vi "PH_Timing.ProcCases.vi"(0 "i ref in":refnum<vi>, 1 "selector":string, 2 "Data":T1, 3 "call cluster":T2={"Object"="", "Selector"="", "CallType"=enum."synchronous", "Async Object"="", "Async Selector"="", "Data Descriptor"="", "Data"=[], "Error #"=0, "Expire"=0}, 5 "error in (no error)":errorcluster) -> (14 "i ref out":refnum<vi>, 17 "answer cluster":T2={"Object"="", "Selector"="", "CallType"=enum."synchronous", "Async Object"="", "Async Selector"="", "Data Descriptor"="", "Data"=[], "Error #"=0, "Expire"=0}, 19 "error out":errorcluster)   [LabVIEW 2014, in "PH_Timing.lvlib"]
doc: "This method is called by a process from within the default case in the event loop. The methods of a class that are linked to events will be called from THIS method. Add your code here."
uses:
  PH_Timing.lvlib
  CS_Core/CSSystem/CoreDefs/CoreDefs.call_type.ctl
  CS_Core/BaseProcess/BaseProcess.descriptor string definition.ctl
  CS_Core/CSSystem/CoreDefs/CoreDefs.rawDataType.ctl
  PH_Timing.Timing Mode.ctl
  PH_Timing.Slow Trigger Settings.ctl
  PH_Timing.Phase FEs.ctl
  PH_Basics/PH_PowerUnit_BaseClass/PH_PowerUnit_BaseClass.SM States.ctl
  CS_Core/CSSystem/CoreLib/CoreLib.byte array 2 short.vi
  CS_Core/CSSystem/CoreLib/CoreLib.string 2 byte array.vi
  CS_Core/CSSystem/CoreLib/CoreLib.byte array 2 double.vi
  CS_Core/CSSystem/CoreLib/CoreLib.byte array 2 string.vi
  CS_Core/CSSystem/CoreLib/CoreLib.byte array 2 int.vi
  CS_Core/BaseProcess/BaseProcess.lvlib
  CS_Core/CSSystem/CoreLib/CoreLib.lvlib
  CS_Core/CAEObj/CAEObj.lvlib
  PH_Basics/PH_Common/PH_Common.lvlib
  PH_Basics/PH_StatusHandler/PH_StatusHandler.lvlib
  PH_Basics/PH_PowerUnit_BaseClass/PH_PowerUnit_BaseClass.lvlib
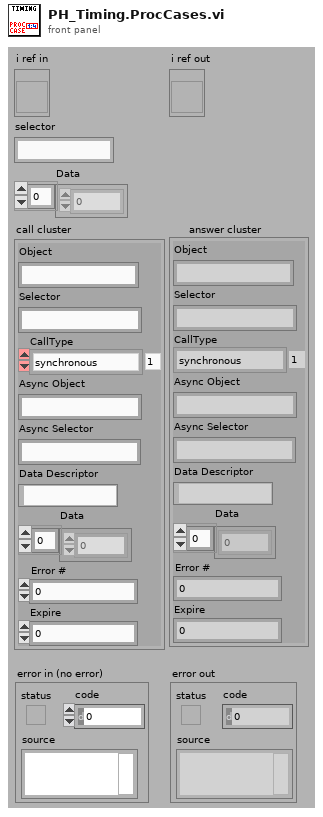
[diagram p1: front panel]
types:
  T1 = typedef "CoreDefs.rawDataType.ctl" = i8[]
  T2 = typedef "CoreDefs.call_type.ctl" = cluster{"Object":string, "Selector":string, "CallType":enum16{"simple", "synchronous", "asynchronous"}, "Async Object":string, "Async Selector":string, "Data Descriptor":T3, "Data":T1, "Error #":i32, "Expire":u32}
  T3 = typedef "BaseProcess.lvlib/BaseProcess.descriptor string definition.ctl" = string
  T4 = typedef "PH_Timing.lvlib/PH_Timing.Timing Mode.ctl" = cluster{"T2":i16, "Modeselector":enum32{"10 Hz", "0.5 Hz", "Shot"}}
  T5 = typedef "PH_Timing.lvlib/PH_Timing.Slow Trigger Settings.ctl" = cluster{"Delay":dbl, "externally triggered?":bool}
  T6 = typedef "PH_Timing.lvlib/PH_Timing.Phase FEs.ctl" = cluster{"Phase":dbl}
  T7 = typedef "PH_PowerUnit_BaseClass.lvlib/PH_PowerUnit_BaseClass.SM States.ctl" = enum16{".", "Stand by", "Switch PU on", "Configure", "Set Default Voltage", "Set STANDBY", "Set READY", "Wait for Shot Cmd", "Open Dump Rods", "Open Ross Relais", "Close Ross Relais", "Switch PSU on", "Switch PSU off", "Charge", "Switch GD Channel on", "Close Dump Rods", "Rods-TO", "RR-TO", "PSU-TO", "Trigger-TO"}
  T8 = typedef "PH_Timing.lvlib/PH_Timing.i attribute.ctl" = cluster{"Sequencer":cluster{"linked?":bool, "Proc State":string, "Ref State":refnum<vi>}, "Gate Generator":cluster{"GD":cluster{"Device Status":T9, "linked?":bool}, "Settings":T10, "GUI Ref":refnum<vi>}, "Interlock Bypass":cluster{"Instancename":string, "Switch linked?":bool, "Device Status":T9, "Ref Status":refnum<vi>}, "Roughtuner":cluster{"Settings":T11, "GUI Ref":refnum<vi>, "GD":cluster{"Device Status":T9, "linked?":bool}}, "0,5Hz Gater":cluster{"Settings":T12, "GUI Ref":refnum<vi>, "GD":cluster{"Device Status":T9, "linked?":bool}}, "Slow Trigger":cluster{"Settings":T5, "GUI Ref":refnum<vi>, "Service ID Delay":i32, "Service ID Ext Trig":i32, "Wanted Settings":T5}, "Timing Mode":cluster{"Mode":T4, "GUI Ref":refnum<vi>, "Service ID T2":i32, "Service ID Mode":i32, "Wanted Mode":T4}, "ns Generator":cluster{"Settings":T13, "ns Generator Settings":refnum<vi>, "GD":cluster{"Device Status":T9, "linked?":bool}}, "Phase FEs":cluster{"Settings":T6, "GUI Ref":refnum<vi>, "Service ID Phase":i32, "Wanted Settings":T6}, "GD GUI Refs":refnum<vi>[], "Heads":T16[], "GUI Ref Delete":refnum<vi>}
  T9 = typedef "PH_StatusHandler.lvlib/PH_StatusHandler.Status.ctl" = i16
  T10 = typedef "PH_Timing.lvlib/PH_Timing.GateGen.ctl" = cluster{"Instance":string, "Channel Gate":i32, "Channel T2":i32, "Width Gate":dbl, "Width T2":dbl, "Delay Gate":dbl, "Delay T2":dbl, "Gate activ":bool, "T2 activ":bool, "System Mode":enum16{"Normal", "Single", "Burst", "Duty Cycle"}}
  T11 = typedef "PH_Timing.lvlib/PH_Timing.Roughtuner.ctl" = cluster{"Instance":string, "Phase PHELIX / UNILAC":cluster{"Channel":u16, "relative to":u16, "Delay [ms]":dbl}, "Pulse Length":cluster{"Channel":u16, "relative to":u16, "Delay [ms]":dbl}, "Trigger":cluster{"externally?":bool, "Rate [Hz]":dbl}}
  T12 = typedef "PH_Timing.lvlib/PH_Timing.0.5HzGater.ctl" = cluster{"Instance":string, "Channel ns FE Delay":i32, "Channel 0.5Hz":i32, "Width ns FE Delay":dbl, "Width 0.5Hz":dbl, "Delay ns FE Delay":dbl, "Delay 0.5Hz":dbl, "ns FE Delay active":bool, "0.5Hz activ":bool, "ns FE Delay inverted":bool, "0.5Hz inverted":bool}
  T13 = typedef "PH_Timing.lvlib/PH_Timing.ns Generator.ctl" = cluster{"Instance":string, "Phase fs / ns FE":cluster{"Channel":T14, "Settings":T15}}
  T14 = typedef "Stanford Research DG645 - Driver.lvlib/Channel.ctl" = i32
  T15 = typedef "PH_SRDG645.lvlib/PH_SRDG645.Channel Settings.ctl" = cluster{"Delay [s]":dbl, "relative to":i32}
  T16 = typedef "PH_Timing.lvlib/PH_Timing.PU Data.ctl" = cluster{"linked?":bool, "Data":T17, "GD":cluster{"Device Status":T9, "linked?":bool}, "GUI Ref":refnum<vi>, "PU":T18}
  T17 = typedef "PH_Timing.lvlib/PH_Timing.PU Info.ctl" = cluster{"Act CH?":bool, "GD":string, "CH":i32, "Delay":dbl, "active":bool, "in Use?":bool}
  T18 = typedef "PH_PP_Common.lvlib/PH_PP_Common.PUs.ctl" = enum16{"no Info", "PA-19mm-1", "PA-19mm-2", "PA-45mm-PILC", "PA-45mm-MAIN", "MA-PU-1", "MA-PU-2", "MA-PU-3", "MA-PU-4", "MA-PU-5", "MA-PU-6", "MA-FR", "MA-PILC", "PA-45mm-DP"}
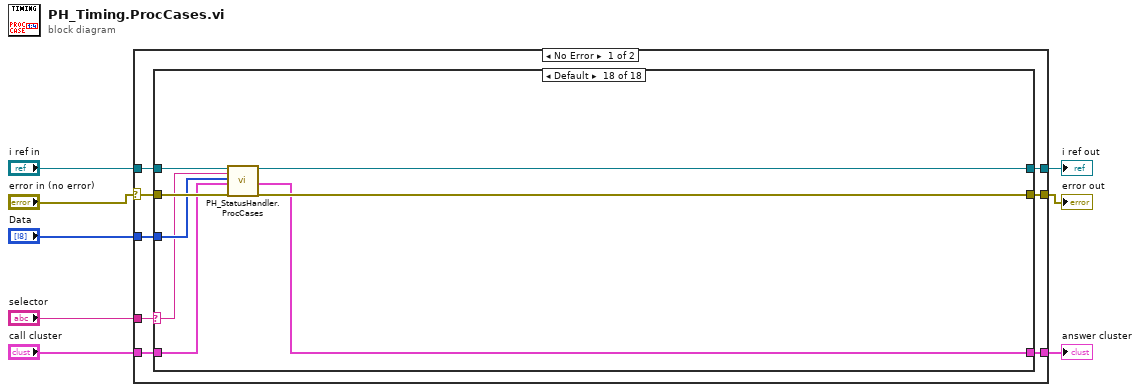
[diagram p0: block diagram]
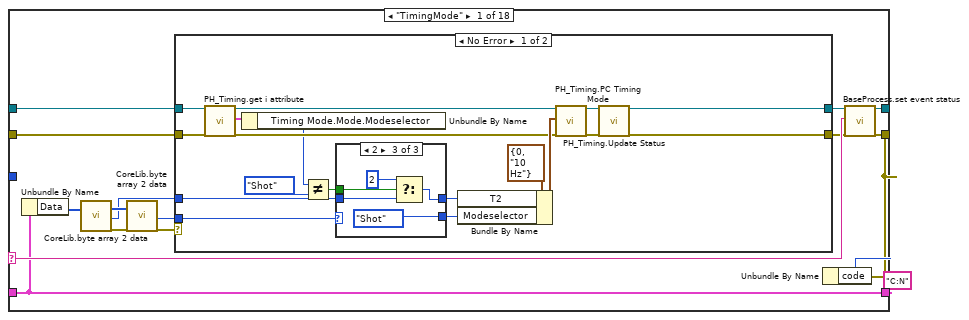
[diagram p2: hidden frame]
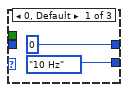
[diagram p3: hidden frame]
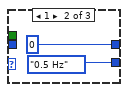
[diagram p4: hidden frame]
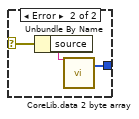
[diagram p6: hidden frame]
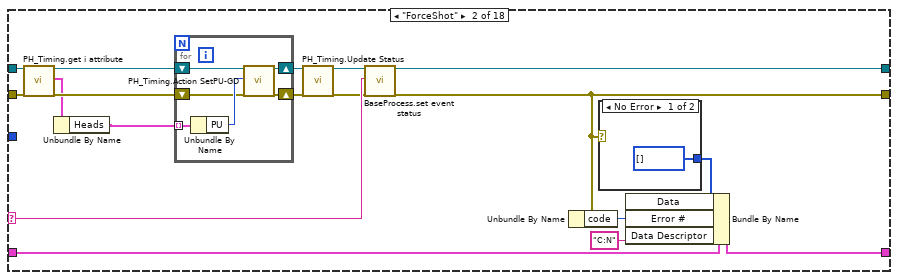
[diagram p7: hidden frame]
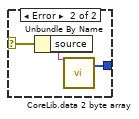
[diagram p8: hidden frame]
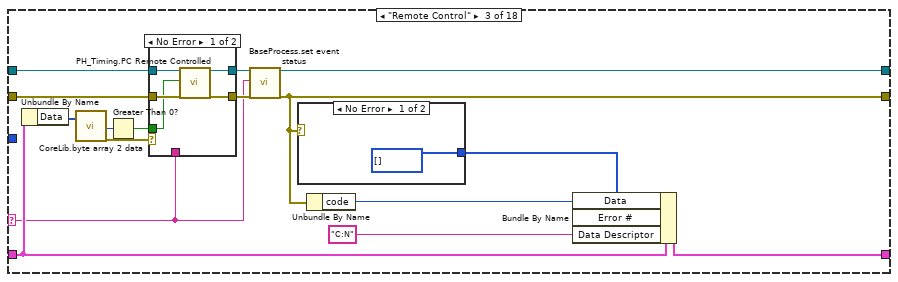
[diagram p9: hidden frame]
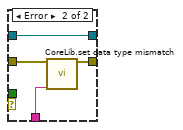
[diagram p10: hidden frame]
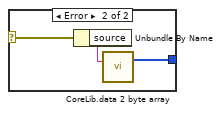
[diagram p11: hidden frame]
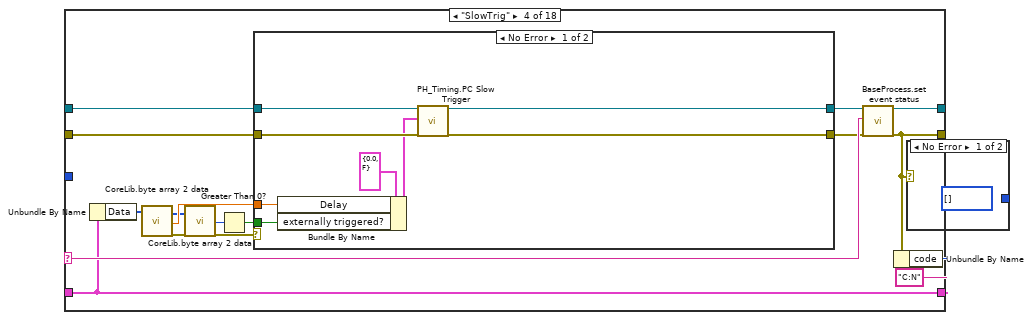
[diagram p12: hidden frame]
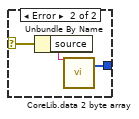
[diagram p14: hidden frame]
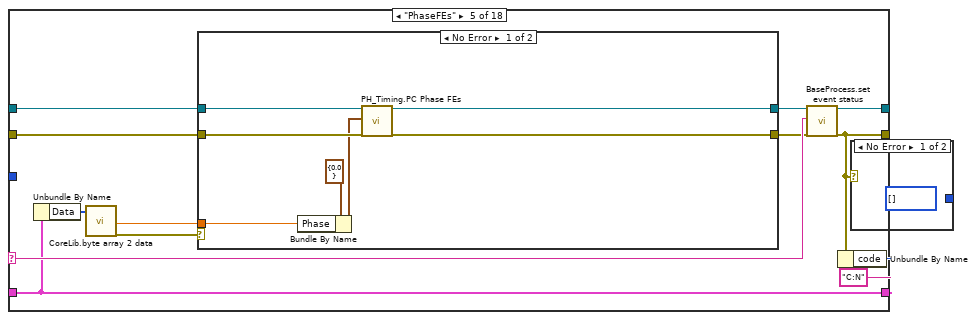
[diagram p15: hidden frame]
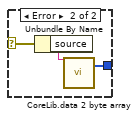
[diagram p17: hidden frame]
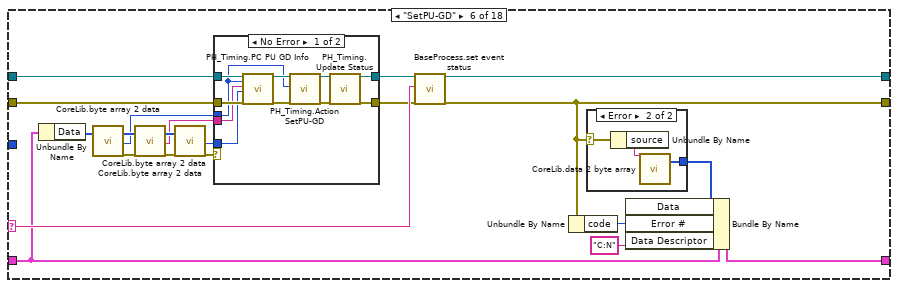
[diagram p18: hidden frame]
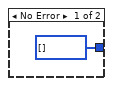
[diagram p20: hidden frame]
diagram:
  n1 = case shown="No Error" "error in (no error)" {
    selector: "error in (no error)" -> [w9 w690]
    tunnel: "selector" -> [w16 _]
    tunnel: [w15 w691] -> w7
    tunnel: "Data" -> [w14 _]
    tunnel: "call cluster" -> [w13 w691]
    tunnel: "i ref in" -> [w12 w692]
    tunnel: [w11 w692] -> w3
    tunnel: [w10 w690] -> w2
    frame No Error {
      n2 = case shown="Default" w16 {
        selector: w16 -> [w28 w79 w96 w137 w166 w200 w235 w267 w317 w351 w386 w444 w500 w534 w568 w602 w641 w683]
        tunnel: w14 -> [_ _ _ _ _ _ _ w259 w311 w345 w378 w436 w494 w528 w562 w594 w633 w684]
        tunnel: w12 -> [w25 w72 w100 w131 w160 w197 w225 w261 w313 w347 w380 w438 w496 w530 w564 w596 w635 w682]
        tunnel: [w30 w81 w107 w139 w168 w202 w237 w270 w320 w354 w389 w447 w503 w537 w571 w605 w630 w689] -> w11
        tunnel: w13 -> [w23 w78 w99 w134 w163 w186 w229 w268 w318 w352 w387 w445 w501 w535 w569 w603 w642 w685]
        tunnel: [w33 w84 w110 w142 w171 w205 w240 w273 w323 w357 w392 w450 w506 w540 w574 w608 w645 w686] -> w15
        tunnel: w9 -> [w24 w71 w101 w132 w161 w196 w226 w260 w312 w346 w379 w437 w495 w529 w563 w595 w634 w688]
        tunnel: [w31 w82 w108 w140 w169 w203 w238 w271 w321 w355 w390 w448 w504 w538 w572 w606 w629 w687] -> w10
        frame "TimingMode" {
          n3 = Unbundle By Name(w23) -> ("Data"=w18:T1)
          n4 = call-poly "CoreLib.byte array 2 data.vi"("byteArray"=w18) -> ("byteArray out"=w20:T1, "i16"=w19:i16, "error out"=w21:errorcluster)  [unwired: 16 in]
          n5 = call-poly "CoreLib.byte array 2 data.vi"("byteArray"=w20, "error in (no error)"=w21) -> ("i16"=w17:i16, "error out"=w22:errorcluster)  [unwired: 15 in, 1 out]
          n6 = case shown="No Error" w22 {
            tunnel: [w37 w63] -> w26
            tunnel: w25 -> [w44 w63]
            tunnel: w24 -> [w52 w62]
            tunnel: [w38 w62] -> w27
            tunnel: w19 -> [w48 _]
            tunnel: w17 -> [w49 _]
            frame No Error {
              n7 = call "PH_Timing.get i attribute.vi"("i ref in"=w44, "error in (no error)"=w52) -> ("i ref out"=w43:refnum<vi>, "i attribute"=w42:T8, "error out"=w45:errorcluster)  [unwired: 15 in]
              n8 = Unbundle By Name(w42) -> ("Timing Mode.Mode.Modeselector"=w41:enum32{"10 Hz", "0.5 Hz", "Shot"})
              n9 = Not Equal?(x=w41, y=enum32{"10 Hz", "0.5 Hz", "Shot"}."Shot") -> (x != y?=w39:bool)
              n10 = case shown="2" w49 {
                tunnel: w48 -> [_ _ w59]
                tunnel: [enum32{"10 Hz", "0.5 Hz", "Shot"}."10 Hz" ("Modeselector") enum32{"10 Hz", "0.5 Hz", "Shot"}."0.5 Hz" ("Modeselector") enum32{"10 Hz", "0.5 Hz", "Shot"}."Shot" ("Modeselector")] -> w47
                tunnel: [i16 0 ("T2 [s]") i16 0 ("T2 [s]") w58] -> w46
                tunnel: w39 -> [_ _ w60]
                frame 0, Default {
                }
                frame 1 {
                }
                frame 2 {
                  n11 = Select(t=i16 2, s=w60, f=w59) -> (s? t:f=w58:i16)
                }
              }
              n12 = Bundle By Name(cluster=T4 {"T2"=0, "Modeselector"=enum."10 Hz"} ("Timing Mode"), "T2"=w46, "Modeselector"=w47) -> (w50:T4)
              n13 = call "PH_Timing.PC Timing Mode.vi"("i ref in"=w43, "Timing Mode"=w50, "error IO"=w45) -> ("i ref out"=w36:refnum<vi>, "error out"=w35:errorcluster)  [unwired: 15 in]
              n14 = call "PH_Timing.Update Status.vi"("i ref in"=w36, "error in (no error)"=w35) -> ("i ref out"=w37:refnum<vi>, "error out"=w38:errorcluster)  [unwired: 16 in]
            }
            frame Error {
            }
          }
          n15 = call "BaseProcess.set event status.vi"("i ref in"=w26, "EventStatus"=w28, "error in (no error)"=w27) -> ("i ref out"=w30:refnum<vi>, "error out"=w31:errorcluster)  [unwired: 14 in, 1 out]
          n16 = Unbundle By Name(w31) -> ("code"=w34:i32)
          n17 = case shown="No Error" w31 {
            selector: w31 -> [_ w67]
            tunnel: [T1 [] ("byteArray out") w66] -> w32
            frame No Error {
            }
            frame Error {
              n18 = Unbundle By Name(w67) -> ("source"=w65:string)
              n19 = call-poly "CoreLib.data 2 byte array.vi"("string"=w65) -> ("byteArray out"=w66:T1)  [unwired: 18 in]
            }
          }
          n20 = Bundle By Name(cluster=w23, "Data"=w32, "Error #"=w34, "Data Descriptor"="C:N") -> (w33:T2)
        }
        frame "ForceShot" {
          n21 = call "PH_Timing.get i attribute.vi"("i ref in"=w72, "error in (no error)"=w71) -> ("i ref out"=w76:refnum<vi>, "i attribute"=w75:T8, "error out"=w77:errorcluster)  [unwired: 15 in]
          n22 = Unbundle By Name(w75) -> ("Heads"=w68:T16[])
          n23 = for {
            shift-right: [w87] -> w73
            shift-left: w76 -> [w89]
            shift-right: [w86] -> w74
            shift-left: w77 -> [w88]
            tunnel: w68 -> [w91] mode=indexing
            n24 = Unbundle By Name(w91) -> ("PU"=w90:T18)
            n25 = call "PH_Timing.Action SetPU-GD.vi"("i ref in"=w89, "PU"=w90, "error in (no error)"=w88) -> ("i ref out"=w87:refnum<vi>, "error out"=w86:errorcluster)  [unwired: 15 in]
          }
          n26 = call "PH_Timing.Update Status.vi"("i ref in"=w73, "error in (no error)"=w74) -> ("i ref out"=w69:refnum<vi>, "error out"=w70:errorcluster)  [unwired: 16 in]
          n27 = call "BaseProcess.set event status.vi"("i ref in"=w69, "EventStatus"=w79, "error in (no error)"=w70) -> ("i ref out"=w81:refnum<vi>, "error out"=w82:errorcluster)  [unwired: 14 in, 1 out]
          n28 = Unbundle By Name(w82) -> ("code"=w85:i32)
          n29 = case shown="No Error" w82 {
            selector: w82 -> [_ w95]
            tunnel: [T1 [] ("byteArray out") w94] -> w83
            frame No Error {
            }
            frame Error {
              n30 = Unbundle By Name(w95) -> ("source"=w93:string)
              n31 = call-poly "CoreLib.data 2 byte array.vi"("string"=w93) -> ("byteArray out"=w94:T1)  [unwired: 18 in]
            }
          }
          n32 = Bundle By Name(cluster=w78, "Data"=w83, "Error #"=w85, "Data Descriptor"="C:N") -> (w84:T2)
        }
        frame "Remote Control" {
          n33 = Unbundle By Name(w99) -> ("Data"=w102:T1)
          n34 = call-poly "CoreLib.byte array 2 data.vi"("byteArray"=w102) -> ("i16"=w103:i16, "error out"=w105:errorcluster)  [unwired: 16 in, 1 out]
          n35 = Greater Than 0?(x=w103) -> (x > 0?=w104:bool)
          n36 = case shown="No Error" w105 {
            tunnel: [w113 w120] -> w98
            tunnel: w100 -> [w115 w120]
            tunnel: w101 -> [w114 w119]
            tunnel: [w116 w118] -> w97
            tunnel: w96 -> [_ w117]
            tunnel: w104 -> [w112 _]
            frame No Error {
              n37 = call "PH_Timing.PC Remote Controlled.vi"("i ref in"=w115, "Remote Controlled?"=w112, "error in (no error)"=w114) -> ("i ref out"=w113:refnum<vi>, "error out"=w116:errorcluster)  [unwired: 15 in]
            }
            frame Error {
              n38 = call "CoreLib.set data type mismatch.vi"("error in (no error)"=w119, "error source"=w117) -> ("error out"=w118:errorcluster)  [unwired: 17 in]
            }
          }
          n39 = call "BaseProcess.set event status.vi"("i ref in"=w98, "EventStatus"=w96, "error in (no error)"=w97) -> ("i ref out"=w107:refnum<vi>, "error out"=w108:errorcluster)  [unwired: 14 in, 1 out]
          n40 = case shown="No Error" w108 {
            selector: w108 -> [_ w124]
            tunnel: [T1 [] ("byteArray out") w123] -> w109
            frame No Error {
            }
            frame Error {
              n41 = Unbundle By Name(w124) -> ("source"=w122:string)
              n42 = call-poly "CoreLib.data 2 byte array.vi"("string"=w122) -> ("byteArray out"=w123:T1)  [unwired: 18 in]
            }
          }
          n43 = Unbundle By Name(w108) -> ("code"=w111:i32)
          n44 = Bundle By Name(cluster=w99, "Data"=w109, "Error #"=w111, "Data Descriptor"="C:N") -> (w110:T2)
        }
        frame "SlowTrig" {
          n45 = Unbundle By Name(w134) -> ("Data"=w130:T1)
          n46 = call-poly "CoreLib.byte array 2 data.vi"("byteArray"=w130) -> ("byteArray out"=w127:T1, "d64"=w133:dbl, "error out"=w129:errorcluster)  [unwired: 16 in]
          n47 = call-poly "CoreLib.byte array 2 data.vi"("byteArray"=w127, "error in (no error)"=w129) -> ("i16"=w126:i16, "error out"=w128:errorcluster)  [unwired: 15 in, 1 out]
          n48 = Greater Than 0?(x=w126) -> (x > 0?=w125:bool)
          n49 = case shown="No Error" w128 {
            tunnel: [w145 w152] -> w135
            tunnel: w132 -> [w150 w153]
            tunnel: [w144 w153] -> w136
            tunnel: w131 -> [w151 w152]
            tunnel: w133 -> [w148 _]
            tunnel: w125 -> [w147 _]
            frame No Error {
              n50 = Bundle By Name(cluster=T5 {"Delay"=0.0, "externally triggered?"=FALSE} ("Slow Trigger Settings"), "Delay"=w148, "externally triggered?"=w147) -> (w146:T5)
              n51 = call "PH_Timing.PC Slow Trigger.vi"("i ref in"=w151, "Slow Trigger Settings"=w146, "error IO"=w150) -> ("i ref out"=w145:refnum<vi>, "error out"=w144:errorcluster)  [unwired: 15 in]
            }
            frame Error {
            }
          }
          n52 = call "BaseProcess.set event status.vi"("i ref in"=w135, "EventStatus"=w137, "error in (no error)"=w136) -> ("i ref out"=w139:refnum<vi>, "error out"=w140:errorcluster)  [unwired: 14 in, 1 out]
          n53 = Unbundle By Name(w140) -> ("code"=w143:i32)
          n54 = case shown="No Error" w140 {
            selector: w140 -> [_ w157]
            tunnel: [T1 [] ("byteArray out") w156] -> w141
            frame No Error {
            }
            frame Error {
              n55 = Unbundle By Name(w157) -> ("source"=w155:string)
              n56 = call-poly "CoreLib.data 2 byte array.vi"("string"=w155) -> ("byteArray out"=w156:T1)  [unwired: 18 in]
            }
          }
          n57 = Bundle By Name(cluster=w134, "Data"=w141, "Error #"=w143, "Data Descriptor"="C:N") -> (w142:T2)
        }
        frame "PhaseFEs" {
          n58 = Unbundle By Name(w163) -> ("Data"=w159:T1)
          n59 = call-poly "CoreLib.byte array 2 data.vi"("byteArray"=w159) -> ("d64"=w162:dbl, "error out"=w158:errorcluster)  [unwired: 16 in, 1 out]
          n60 = case shown="No Error" w158 {
            tunnel: [w175 w180] -> w164
            tunnel: w161 -> [w178 w181]
            tunnel: [w174 w181] -> w165
            tunnel: w160 -> [w179 w180]
            tunnel: w162 -> [w176 _]
            frame No Error {
              n61 = Bundle By Name(cluster=T6 {"Phase"=0.0} ("FE Phase"), "Phase"=w176) -> (w173:T6)
              n62 = call "PH_Timing.PC Phase FEs.vi"("i ref in"=w179, "FE Phase"=w173, "error IO"=w178) -> ("i ref out"=w175:refnum<vi>, "error out"=w174:errorcluster)  [unwired: 15 in]
            }
            frame Error {
            }
          }
          n63 = call "BaseProcess.set event status.vi"("i ref in"=w164, "EventStatus"=w166, "error in (no error)"=w165) -> ("i ref out"=w168:refnum<vi>, "error out"=w169:errorcluster)  [unwired: 14 in, 1 out]
          n64 = Unbundle By Name(w169) -> ("code"=w172:i32)
          n65 = case shown="No Error" w169 {
            selector: w169 -> [_ w185]
            tunnel: [T1 [] ("byteArray out") w184] -> w170
            frame No Error {
            }
            frame Error {
              n66 = Unbundle By Name(w185) -> ("source"=w183:string)
              n67 = call-poly "CoreLib.data 2 byte array.vi"("string"=w183) -> ("byteArray out"=w184:T1)  [unwired: 18 in]
            }
          }
          n68 = Bundle By Name(cluster=w163, "Data"=w170, "Error #"=w172, "Data Descriptor"="C:N") -> (w171:T2)
        }
        frame "SetPU-GD" {
          n69 = Unbundle By Name(w186) -> ("Data"=w195:T1)
          n70 = call-poly "CoreLib.byte array 2 data.vi"("byteArray"=w195) -> ("byteArray out"=w193:T1, "i16"=w189:i16, "error out"=w194:errorcluster)  [unwired: 16 in]
          n71 = call-poly "CoreLib.byte array 2 data.vi"("byteArray"=w193, "error in (no error)"=w194) -> ("byteArray out"=w190:T1, "string"=w188:string, "error out"=w192:errorcluster)  [unwired: 15 in]
          n72 = call-poly "CoreLib.byte array 2 data.vi"("byteArray"=w190, "error in (no error)"=w192) -> ("i32"=w187:i32, "error out"=w191:errorcluster)  [unwired: 15 in, 1 out]
          n73 = case shown="No Error" w191 {
            tunnel: [w208 w219] -> w198
            tunnel: w197 -> [w217 w219]
            tunnel: w196 -> [w216 w218]
            tunnel: [w209 w218] -> w199
            tunnel: w189 -> [w207 _]
            tunnel: w188 -> [w215 _]
            tunnel: w187 -> [w212 _]
            frame No Error {
              n74 = call "PH_Timing.PC PU GD Info.vi"("i ref in"=w217, "PU"=w207, "GD Instance Name"=w215, "PU Channel"=w212, "error in"=w216) -> ("i ref out"=w211:refnum<vi>, "error out"=w210:errorcluster)  [unwired: 13 in]
              n75 = call "PH_Timing.Action SetPU-GD.vi"("i ref in"=w211, "PU"=w207, "error in (no error)"=w210) -> ("i ref out"=w214:refnum<vi>, "error out"=w213:errorcluster)  [unwired: 15 in]
              n76 = call "PH_Timing.Update Status.vi"("i ref in"=w214, "error in (no error)"=w213) -> ("i ref out"=w208:refnum<vi>, "error out"=w209:errorcluster)  [unwired: 16 in]
            }
            frame Error {
            }
          }
          n77 = call "BaseProcess.set event status.vi"("i ref in"=w198, "EventStatus"=w200, "error in (no error)"=w199) -> ("i ref out"=w202:refnum<vi>, "error out"=w203:errorcluster)  [unwired: 14 in, 1 out]
          n78 = Unbundle By Name(w203) -> ("code"=w206:i32)
          n79 = case shown="Error" w203 {
            selector: w203 -> [_ w223]
            tunnel: [T1 [] ("byteArray out") w222] -> w204
            frame No Error {
            }
            frame Error {
              n80 = Unbundle By Name(w223) -> ("source"=w221:string)
              n81 = call-poly "CoreLib.data 2 byte array.vi"("string"=w221) -> ("byteArray out"=w222:T1)  [unwired: 18 in]
            }
          }
          n82 = Bundle By Name(cluster=w186, "Data"=w204, "Error #"=w206, "Data Descriptor"="C:N") -> (w205:T2)
        }
        frame "SetPUDelay" {
          n83 = Unbundle By Name(w229) -> ("Data"=w232:T1)
          n84 = call-poly "CoreLib.byte array 2 data.vi"("byteArray"=w232) -> ("byteArray out"=w228:T1, "i16"=w224:i16, "error out"=w231:errorcluster)  [unwired: 16 in]
          n85 = call-poly "CoreLib.byte array 2 data.vi"("byteArray"=w228, "error in (no error)"=w231) -> ("d64"=w227:dbl, "error out"=w230:errorcluster)  [unwired: 15 in, 1 out]
          n86 = case shown="No Error" w230 {
            tunnel: [w243 w252] -> w233
            tunnel: w226 -> [w251 w253]
            tunnel: [w246 w253] -> w234
            tunnel: w225 -> [w249 w252]
            tunnel: w227 -> [w250 _]
            tunnel: w224 -> [w242 _]
            frame No Error {
              n87 = call "PH_Timing.PC PU Delay.vi"("i ref in"=w249, "PU"=w242, "PU Delay"=w250, "error in"=w251) -> ("i ref out"=w244:refnum<vi>, "error out"=w247:errorcluster)  [unwired: 14 in]
              n88 = call "PH_Timing.Action SetPU-GD.vi"("i ref in"=w244, "PU"=w242, "error in (no error)"=w247) -> ("i ref out"=w245:refnum<vi>, "error out"=w248:errorcluster)  [unwired: 15 in]
              n89 = call "PH_Timing.Update Status.vi"("i ref in"=w245, "error in (no error)"=w248) -> ("i ref out"=w243:refnum<vi>, "error out"=w246:errorcluster)  [unwired: 16 in]
            }
            frame Error {
            }
          }
          n90 = call "BaseProcess.set event status.vi"("i ref in"=w233, "EventStatus"=w235, "error in (no error)"=w234) -> ("i ref out"=w237:refnum<vi>, "error out"=w238:errorcluster)  [unwired: 14 in, 1 out]
          n91 = Unbundle By Name(w238) -> ("code"=w241:i32)
          n92 = case shown="No Error" w238 {
            selector: w238 -> [_ w257]
            tunnel: [T1 [] ("byteArray out") w256] -> w239
            frame No Error {
            }
            frame Error {
              n93 = Unbundle By Name(w257) -> ("source"=w255:string)
              n94 = call-poly "CoreLib.data 2 byte array.vi"("string"=w255) -> ("byteArray out"=w256:T1)  [unwired: 18 in]
            }
          }
          n95 = Bundle By Name(cluster=w229, "Data"=w239, "Error #"=w241, "Data Descriptor"="C:N") -> (w240:T2)
        }
        frame "_StatusInterlockSwitch" {
          n96 = call "CAEObj.unfold trend data.vi"("i ref in"=w261, "raw trend data"=w259) -> ("no link"=w265:bool, "data"=w264:i8[], "typeDescriptor"=w258:string, "error out"=w266:errorcluster)  [unwired: 9 in, 5 out]
          n97 = case shown="No Error" w266 {
            tunnel: [w293 w302] -> w262
            tunnel: w261 -> [w287 w302]
            tunnel: w260 -> [w289 w301]
            tunnel: [w294 w301] -> w263
            tunnel: w265 -> [w276 _]
            tunnel: w264 -> [w292 _]
            tunnel: w258 -> [w290 _]
            frame No Error {
              n98 = call "PH_Timing.get i attribute.vi"("i ref in"=w287, "error in (no error)"=w289) -> ("i ref out"=w286:refnum<vi>, "i attribute"=w281:T8, "error out"=w288:errorcluster)  [unwired: 15 in]
              n99 = call "PH_StatusHandler.get Status DIM Service.vi"("no link"=w276, "typeDescriptor"=w290, "data"=w292) -> ("Status"=w291:T9)  [unwired: 1 in]
              n100 = Unbundle By Name(w281) -> ("Interlock Bypass.Switch linked?"=w280:bool)
              n101 = Not(x=w276) -> (.not. x?=w275:bool)
              n102 = call "PH_Timing.PC Status Interlockswitch.vi"("i ref in"=w286, "IL Switch Status"=w291, "no link"=w276, "error in"=w288) -> ("i ref out"=w285:refnum<vi>, "error out"=w283:errorcluster)  [unwired: 14 in]
              n103 = Bundle("Switch linked?"=w280, w275) -> (w279:cluster{"Switch linked?":bool, bool})  [unwired: 1 in]
              n104 = Equal?(x=w279, y=cluster{"linked?":bool, "no link":bool} {"linked?"=FALSE, "no link"=TRUE}) -> (x = y?=w277:bool)
              n105 = case shown="True" w277 {
                tunnel: w285 -> [w296 w300]
                tunnel: [w296 w299] -> w284
                tunnel: w283 -> [w295 w298]
                tunnel: [w295 w297] -> w282
                frame False {
                }
                frame True {
                  n106 = call "PH_Timing.Action Switch Interlock Bypass.vi"("i ref in"=w300, "error in (no error)"=w298) -> ("i ref out"=w299:refnum<vi>, "error out"=w297:errorcluster)  [unwired: 16 in]
                }
              }
              n107 = call "PH_Timing.Update Status.vi"("i ref in"=w284, "error in (no error)"=w282) -> ("i ref out"=w293:refnum<vi>, "error out"=w294:errorcluster)  [unwired: 16 in]
            }
            frame Error {
            }
          }
          n108 = call "BaseProcess.set event status.vi"("i ref in"=w262, "EventStatus"=w267, "error in (no error)"=w263) -> ("i ref out"=w270:refnum<vi>, "error out"=w271:errorcluster)  [unwired: 14 in, 1 out]
          n109 = Unbundle By Name(w271) -> ("code"=w274:i32)
          n110 = case shown="No Error" w271 {
            selector: w271 -> [_ w306]
            tunnel: [T1 [] ("byteArray out") w305] -> w272
            frame No Error {
            }
            frame Error {
              n111 = Unbundle By Name(w306) -> ("source"=w304:string)
              n112 = call-poly "CoreLib.data 2 byte array.vi"("string"=w304) -> ("byteArray out"=w305:T1)  [unwired: 18 in]
            }
          }
          n113 = Bundle By Name(cluster=w268, "Data"=w272, "Error #"=w274, "Data Descriptor"="C:N") -> (w273:T2)
        }
        frame "_linkBNCChannelInfo" {
          n114 = call "CAEObj.unfold trend data.vi"("i ref in"=w313, "raw trend data"=w311) -> ("no link"=w315:bool, "data"=w314:i8[], "serviceName"=w310:string, "typeDescriptor"=w309:string, "error out"=w316:errorcluster)  [unwired: 9 in, 4 out]
          n115 = case shown="No Error" w316 {
            tunnel: [w327 w336] -> w308
            tunnel: w313 -> [w333 w336]
            tunnel: w312 -> [w334 w335]
            tunnel: [w325 w335] -> w307
            tunnel: w315 -> [w332 _]
            tunnel: w314 -> [w331 _]
            tunnel: w310 -> [w330 _]
            tunnel: w309 -> [w329 _]
            frame No Error {
              n116 = call "PH_Timing.PC link BNC Channel Infos.vi"("i ref in"=w333, "data"=w331, "Service Name"=w330, "typeDescriptor"=w329, "no link"=w332, "error in"=w334) -> ("i ref out"=w328:refnum<vi>, "error out"=w326:errorcluster)  [unwired: 12 in]
              n117 = call "PH_Timing.Update Status.vi"("i ref in"=w328, "error in (no error)"=w326) -> ("i ref out"=w327:refnum<vi>, "error out"=w325:errorcluster)  [unwired: 16 in]
            }
            frame Error {
            }
          }
          n118 = call "BaseProcess.set event status.vi"("i ref in"=w308, "EventStatus"=w317, "error in (no error)"=w307) -> ("i ref out"=w320:refnum<vi>, "error out"=w321:errorcluster)  [unwired: 14 in, 1 out]
          n119 = Unbundle By Name(w321) -> ("code"=w324:i32)
          n120 = case shown="No Error" w321 {
            selector: w321 -> [_ w340]
            tunnel: [T1 [] ("byteArray out") w339] -> w322
            frame No Error {
            }
            frame Error {
              n121 = Unbundle By Name(w340) -> ("source"=w338:string)
              n122 = call-poly "CoreLib.data 2 byte array.vi"("string"=w338) -> ("byteArray out"=w339:T1)  [unwired: 18 in]
            }
          }
          n123 = Bundle By Name(cluster=w318, "Data"=w322, "Error #"=w324, "Data Descriptor"="C:N") -> (w323:T2)
        }
        frame "_linkBNCSysModeInfo" {
          n124 = call "CAEObj.unfold trend data.vi"("i ref in"=w347, "raw trend data"=w345) -> ("no link"=w349:bool, "data"=w348:i8[], "serviceName"=w344:string, "typeDescriptor"=w343:string, "error out"=w350:errorcluster)  [unwired: 9 in, 4 out]
          n125 = case shown="No Error" w350 {
            tunnel: [w361 w370] -> w342
            tunnel: w347 -> [w367 w370]
            tunnel: w346 -> [w368 w369]
            tunnel: [w359 w369] -> w341
            tunnel: w349 -> [w366 _]
            tunnel: w348 -> [w365 _]
            tunnel: w344 -> [w364 _]
            tunnel: w343 -> [w363 _]
            frame No Error {
              n126 = call "PH_Timing.PC link BNC System Mode Infos.vi"("i ref in"=w367, "data"=w365, "Service Name"=w364, "typeDescriptor"=w363, "no link"=w366, "error in"=w368) -> ("i ref out"=w362:refnum<vi>, "error out"=w360:errorcluster)  [unwired: 12 in]
              n127 = call "PH_Timing.Update Status.vi"("i ref in"=w362, "error in (no error)"=w360) -> ("i ref out"=w361:refnum<vi>, "error out"=w359:errorcluster)  [unwired: 16 in]
            }
            frame Error {
            }
          }
          n128 = call "BaseProcess.set event status.vi"("i ref in"=w342, "EventStatus"=w351, "error in (no error)"=w341) -> ("i ref out"=w354:refnum<vi>, "error out"=w355:errorcluster)  [unwired: 14 in, 1 out]
          n129 = Unbundle By Name(w355) -> ("code"=w358:i32)
          n130 = case shown="No Error" w355 {
            selector: w355 -> [_ w374]
            tunnel: [T1 [] ("byteArray out") w373] -> w356
            frame No Error {
            }
            frame Error {
              n131 = Unbundle By Name(w374) -> ("source"=w372:string)
              n132 = call-poly "CoreLib.data 2 byte array.vi"("string"=w372) -> ("byteArray out"=w373:T1)  [unwired: 18 in]
            }
          }
          n133 = Bundle By Name(cluster=w352, "Data"=w356, "Error #"=w358, "Data Descriptor"="C:N") -> (w357:T2)
        }
        frame "_activateCHs" {
          n134 = call "CAEObj.unfold trend data.vi"("i ref in"=w380, "raw trend data"=w378) -> ("quality"=w375:i32, "no link"=w384:bool, "data"=w383:i8[], "serviceName"=w377:string, "typeDescriptor"=w376:string, "error out"=w385:errorcluster)  [unwired: 9 in, 3 out]
          n135 = case shown="No Error" w385 {
            tunnel: [w403 w428] -> w381
            tunnel: w380 -> [w406 w428]
            tunnel: w379 -> [w405 w427]
            tunnel: [w404 w427] -> w382
            tunnel: w384 -> [w402 _]
            tunnel: w383 -> [w411 _]
            tunnel: w377 -> [w409 _]
            tunnel: w376 -> [w412 _]
            tunnel: w375 -> [w410 _]
            frame No Error {
              n136 = call "PH_DIM.get String.vi"("no link"=w402, "typeDescriptor"=w412, "data"=w411, "quality"=w410) -> ("Output String"=w397:string)
              n137 = call "PH_Strings.Remove trailing Zeros.vi"("Input String"=w397) -> ("Output String"=w396:string)
              n138 = call "PH_PowerUnit_BaseClass.String to SM State.vi"("SM State String"=w396) -> ("SM State"=w395:T7)
              n139 = Equal?(x=w395, y=PH_PowerUnit_BaseClass.SM_States."Switch GD Channel on" ("SM State")) -> (x = y?=w398:bool)
              n140 = call "PH_Timing.PC activate CHs.vi"("i ref in"=w406, "Service Name"=w409, "Activate CH?"=w398, "no link"=w402, "error in"=w405) -> ("i ref out"=w408:refnum<vi>, "PU"=w401:T18, "error out"=w407:errorcluster)  [unwired: 12 in]
              n141 = case shown="False" w402 {
                tunnel: w408 -> [w417 w426]
                tunnel: [w414 w426] -> w400
                tunnel: w407 -> [w416 w425]
                tunnel: [w415 w425] -> w399
                tunnel: w401 -> [w413 _]
                frame False {
                  n142 = case shown="Default" w413 {
                    selector: w413 -> [_ w420]
                    tunnel: w417 -> [w419 w424]
                    tunnel: w416 -> [w418 w423]
                    tunnel: [w418 w422] -> w415
                    tunnel: [w419 w421] -> w414
                    frame "no Info" {
                    }
                    frame Default {
                      n143 = call "PH_Timing.Action link PUs.vi"("i ref in"=w424, "PU index"=w420, "error in (no error)"=w423) -> ("i ref out"=w421:refnum<vi>, "error out"=w422:errorcluster)  [unwired: 15 in]
                    }
                  }
                }
                frame True {
                }
              }
              n144 = call "PH_Timing.Update Status.vi"("i ref in"=w400, "error in (no error)"=w399) -> ("i ref out"=w403:refnum<vi>, "error out"=w404:errorcluster)  [unwired: 16 in]
            }
            frame Error {
            }
          }
          n145 = call "BaseProcess.set event status.vi"("i ref in"=w381, "EventStatus"=w386, "error in (no error)"=w382) -> ("i ref out"=w389:refnum<vi>, "error out"=w390:errorcluster)  [unwired: 14 in, 1 out]
          n146 = Unbundle By Name(w390) -> ("code"=w393:i32)
          n147 = case shown="No Error" w390 {
            selector: w390 -> [_ w432]
            tunnel: [T1 [] ("byteArray out") w431] -> w391
            frame No Error {
            }
            frame Error {
              n148 = Unbundle By Name(w432) -> ("source"=w430:string)
              n149 = call-poly "CoreLib.data 2 byte array.vi"("string"=w430) -> ("byteArray out"=w431:T1)  [unwired: 18 in]
            }
          }
          n150 = Bundle By Name(cluster=w387, "Data"=w391, "Error #"=w393, "Data Descriptor"="C:N") -> (w392:T2)
        }
        frame "_PUsinUse" {
          n151 = call "CAEObj.unfold trend data.vi"("i ref in"=w438, "raw trend data"=w436) -> ("quality"=w434:i32, "no link"=w442:bool, "data"=w441:i8[], "serviceName"=w433:string, "typeDescriptor"=w435:string, "error out"=w443:errorcluster)  [unwired: 9 in, 3 out]
          n152 = case shown="No Error" w443 {
            tunnel: [w464 w485] -> w439
            tunnel: w438 -> [w461 w485]
            tunnel: w437 -> [w460 w484]
            tunnel: [w465 w484] -> w440
            tunnel: w442 -> [w452 _]
            tunnel: w441 -> [w467 _]
            tunnel: w435 -> [w468 _]
            tunnel: w434 -> [w466 _]
            tunnel: w433 -> [w459 _]
            frame No Error {
              n153 = call "PH_DIM.get Boolean.vi"("no link"=w452, "typeDescriptor"=w468, "data"=w467, "quality"=w466) -> ("Value"=w463:i32)
              n154 = Equal?(x=2, y=w463) -> (x = y?=w458:bool)
              n155 = call "PH_Timing.PC PU in Use.vi"("i ref in"=w461, "Service Name"=w459, "PU in Use?"=w458, "no link?"=w452, "error in"=w460) -> ("i ref out"=w456:refnum<vi>, "PU"=w453:T18, "error out"=w457:errorcluster)  [unwired: 12 in]
              n156 = case shown="Default" w453 {
                selector: w453 -> [_ w471]
                tunnel: w456 -> [w470 w475]
                tunnel: w457 -> [w469 w474]
                tunnel: [w470 w473] -> w455
                tunnel: [w469 w472] -> w454
                frame "no Info" {
                }
                frame Default {
                  n157 = call "PH_Timing.Action SetPU-GD.vi"("i ref in"=w475, "PU"=w471, "error in (no error)"=w474) -> ("i ref out"=w473:refnum<vi>, "error out"=w472:errorcluster)  [unwired: 15 in]
                }
              }
              n158 = case shown="\"MA-FR\"" w453 {
                tunnel: [w476 w483] -> w465
                tunnel: [w477 w482] -> w464
                tunnel: w455 -> [w477 w479]
                tunnel: w454 -> [w476 w478]
                frame Default {
                }
                frame "MA-FR" {
                  n159 = call "PH_Timing.Action Switch Interlock Bypass.vi"("i ref in"=w479, "error in (no error)"=w478) -> ("i ref out"=w481:refnum<vi>, "error out"=w480:errorcluster)  [unwired: 16 in]
                  n160 = call "PH_Timing.Update Status.vi"("i ref in"=w481, "error in (no error)"=w480) -> ("i ref out"=w482:refnum<vi>, "error out"=w483:errorcluster)  [unwired: 16 in]
                }
              }
            }
            frame Error {
            }
          }
          n161 = call "BaseProcess.set event status.vi"("i ref in"=w439, "EventStatus"=w444, "error in (no error)"=w440) -> ("i ref out"=w447:refnum<vi>, "error out"=w448:errorcluster)  [unwired: 14 in, 1 out]
          n162 = Unbundle By Name(w448) -> ("code"=w451:i32)
          n163 = case shown="No Error" w448 {
            selector: w448 -> [_ w489]
            tunnel: [T1 [] ("byteArray out") w488] -> w449
            frame No Error {
            }
            frame Error {
              n164 = Unbundle By Name(w489) -> ("source"=w487:string)
              n165 = call-poly "CoreLib.data 2 byte array.vi"("string"=w487) -> ("byteArray out"=w488:T1)  [unwired: 18 in]
            }
          }
          n166 = Bundle By Name(cluster=w445, "Data"=w449, "Error #"=w451, "Data Descriptor"="C:N") -> (w450:T2)
        }
        frame "_linkSRDGChannelInfo" {
          n167 = call "CAEObj.unfold trend data.vi"("i ref in"=w496, "raw trend data"=w494) -> ("no link"=w498:bool, "data"=w497:i8[], "serviceName"=w493:string, "typeDescriptor"=w492:string, "error out"=w499:errorcluster)  [unwired: 9 in, 4 out]
          n168 = case shown="No Error" w499 {
            tunnel: [w510 w519] -> w491
            tunnel: w496 -> [w516 w519]
            tunnel: w495 -> [w517 w518]
            tunnel: [w508 w518] -> w490
            tunnel: w498 -> [w515 _]
            tunnel: w497 -> [w514 _]
            tunnel: w493 -> [w513 _]
            tunnel: w492 -> [w512 _]
            frame No Error {
              n169 = call "PH_Timing.PC link SRDG Channel Infos.vi"("i ref in"=w516, "data"=w514, "Service Name"=w513, "typeDescriptor"=w512, "no link"=w515, "error in"=w517) -> ("i ref out"=w511:refnum<vi>, "error out"=w509:errorcluster)  [unwired: 12 in]
              n170 = call "PH_Timing.Update Status.vi"("i ref in"=w511, "error in (no error)"=w509) -> ("i ref out"=w510:refnum<vi>, "error out"=w508:errorcluster)  [unwired: 16 in]
            }
            frame Error {
            }
          }
          n171 = call "BaseProcess.set event status.vi"("i ref in"=w491, "EventStatus"=w500, "error in (no error)"=w490) -> ("i ref out"=w503:refnum<vi>, "error out"=w504:errorcluster)  [unwired: 14 in, 1 out]
          n172 = Unbundle By Name(w504) -> ("code"=w507:i32)
          n173 = case shown="No Error" w504 {
            selector: w504 -> [_ w523]
            tunnel: [T1 [] ("byteArray out") w522] -> w505
            frame No Error {
            }
            frame Error {
              n174 = Unbundle By Name(w523) -> ("source"=w521:string)
              n175 = call-poly "CoreLib.data 2 byte array.vi"("string"=w521) -> ("byteArray out"=w522:T1)  [unwired: 18 in]
            }
          }
          n176 = Bundle By Name(cluster=w501, "Data"=w505, "Error #"=w507, "Data Descriptor"="C:N") -> (w506:T2)
        }
        frame "_linkSRDGRatelInfo" {
          n177 = call "CAEObj.unfold trend data.vi"("i ref in"=w530, "raw trend data"=w528) -> ("no link"=w532:bool, "data"=w531:i8[], "serviceName"=w527:string, "typeDescriptor"=w526:string, "error out"=w533:errorcluster)  [unwired: 9 in, 4 out]
          n178 = case shown="No Error" w533 {
            tunnel: [w544 w553] -> w525
            tunnel: w530 -> [w550 w553]
            tunnel: w529 -> [w551 w552]
            tunnel: [w542 w552] -> w524
            tunnel: w532 -> [w549 _]
            tunnel: w531 -> [w548 _]
            tunnel: w527 -> [w547 _]
            tunnel: w526 -> [w546 _]
            frame No Error {
              n179 = call "PH_Timing.PC link SRDG Rate Info.vi"("i ref in"=w550, "data"=w548, "Service Name"=w547, "typeDescriptor"=w546, "no link"=w549, "error in"=w551) -> ("i ref out"=w545:refnum<vi>, "error out"=w543:errorcluster)  [unwired: 12 in]
              n180 = call "PH_Timing.Update Status.vi"("i ref in"=w545, "error in (no error)"=w543) -> ("i ref out"=w544:refnum<vi>, "error out"=w542:errorcluster)  [unwired: 16 in]
            }
            frame Error {
            }
          }
          n181 = call "BaseProcess.set event status.vi"("i ref in"=w525, "EventStatus"=w534, "error in (no error)"=w524) -> ("i ref out"=w537:refnum<vi>, "error out"=w538:errorcluster)  [unwired: 14 in, 1 out]
          n182 = Unbundle By Name(w538) -> ("code"=w541:i32)
          n183 = case shown="No Error" w538 {
            selector: w538 -> [_ w557]
            tunnel: [T1 [] ("byteArray out") w556] -> w539
            frame No Error {
            }
            frame Error {
              n184 = Unbundle By Name(w557) -> ("source"=w555:string)
              n185 = call-poly "CoreLib.data 2 byte array.vi"("string"=w555) -> ("byteArray out"=w556:T1)  [unwired: 18 in]
            }
          }
          n186 = Bundle By Name(cluster=w535, "Data"=w539, "Error #"=w541, "Data Descriptor"="C:N") -> (w540:T2)
        }
        frame "_linkSRDG645ChannelInfo" {
          n187 = call "CAEObj.unfold trend data.vi"("i ref in"=w564, "raw trend data"=w562) -> ("no link"=w566:bool, "data"=w565:i8[], "serviceName"=w561:string, "typeDescriptor"=w560:string, "error out"=w567:errorcluster)  [unwired: 9 in, 4 out]
          n188 = case shown="No Error" w567 {
            tunnel: [w577 w587] -> w559
            tunnel: w564 -> [w584 w587]
            tunnel: w563 -> [w585 w586]
            tunnel: [w576 w586] -> w558
            tunnel: w566 -> [w583 _]
            tunnel: w565 -> [w582 _]
            tunnel: w561 -> [w581 _]
            tunnel: w560 -> [w580 _]
            frame No Error {
              n189 = call "PH_Timing.PC link SRDG 645 Channel Infos.vi"("i ref in"=w584, "data"=w582, "Service Name"=w581, "typeDescriptor"=w580, "no link"=w583, "error in"=w585) -> ("i ref out"=w578:refnum<vi>, "error out"=w579:errorcluster)  [unwired: 12 in]
              n190 = call "PH_Timing.Update Status.vi"("i ref in"=w578, "error in (no error)"=w579) -> ("i ref out"=w577:refnum<vi>, "error out"=w576:errorcluster)  [unwired: 16 in]
            }
            frame Error {
            }
          }
          n191 = call "BaseProcess.set event status.vi"("i ref in"=w559, "EventStatus"=w568, "error in (no error)"=w558) -> ("i ref out"=w571:refnum<vi>, "error out"=w572:errorcluster)  [unwired: 14 in, 1 out]
          n192 = Unbundle By Name(w572) -> ("code"=w575:i32)
          n193 = case shown="No Error" w572 {
            selector: w572 -> [_ w591]
            tunnel: [T1 [] ("byteArray out") w590] -> w573
            frame No Error {
            }
            frame Error {
              n194 = Unbundle By Name(w591) -> ("source"=w589:string)
              n195 = call-poly "CoreLib.data 2 byte array.vi"("string"=w589) -> ("byteArray out"=w590:T1)  [unwired: 18 in]
            }
          }
          n196 = Bundle By Name(cluster=w569, "Data"=w573, "Error #"=w575, "Data Descriptor"="C:N") -> (w574:T2)
        }
        frame "_GDStati" {
          n197 = call "CAEObj.unfold trend data.vi"("i ref in"=w596, "raw trend data"=w594) -> ("no link"=w600:bool, "data"=w599:i8[], "serviceName"=w593:string, "typeDescriptor"=w592:string, "error out"=w601:errorcluster)  [unwired: 9 in, 4 out]
          n198 = case shown="No Error" w601 {
            tunnel: [w617 w624] -> w597
            tunnel: w596 -> [w614 w624]
            tunnel: w595 -> [w613 w623]
            tunnel: [w616 w623] -> w598
            tunnel: w600 -> [w618 _]
            tunnel: w599 -> [w621 _]
            tunnel: w593 -> [w622 _]
            tunnel: w592 -> [w619 _]
            frame No Error {
              n199 = call "PH_StatusHandler.get Status DIM Service.vi"("no link"=w618, "typeDescriptor"=w619, "data"=w621) -> ("Status"=w620:T9)  [unwired: 1 in]
              n200 = call "PH_Timing.PC link GDs.vi"("i ref in"=w614, "Service Name"=w622, "no link"=w618, "Status"=w620, "error in"=w613) -> ("i ref out"=w611:refnum<vi>, "error out"=w615:errorcluster)  [unwired: 13 in]
              n201 = call "PH_Timing.set GD Stati to GUI.vi"("VI in"=w611, "error in (no error)"=w615) -> ("VI out"=w610:refnum<vi>, "error out"=w612:errorcluster)  [unwired: 16 in]
              n202 = call "PH_Timing.Update Status.vi"("i ref in"=w610, "error in (no error)"=w612) -> ("i ref out"=w617:refnum<vi>, "error out"=w616:errorcluster)  [unwired: 16 in]
            }
            frame Error {
            }
          }
          n203 = call "BaseProcess.set event status.vi"("i ref in"=w597, "EventStatus"=w602, "error in (no error)"=w598) -> ("i ref out"=w605:refnum<vi>, "error out"=w606:errorcluster)  [unwired: 14 in, 1 out]
          n204 = Unbundle By Name(w606) -> ("code"=w609:i32)
          n205 = case shown="No Error" w606 {
            selector: w606 -> [_ w628]
            tunnel: [T1 [] ("byteArray out") w627] -> w607
            frame No Error {
            }
            frame Error {
              n206 = Unbundle By Name(w628) -> ("source"=w626:string)
              n207 = call-poly "CoreLib.data 2 byte array.vi"("string"=w626) -> ("byteArray out"=w627:T1)  [unwired: 18 in]
            }
          }
          n208 = Bundle By Name(cluster=w603, "Data"=w607, "Error #"=w609, "Data Descriptor"="C:N") -> (w608:T2)
        }
        frame "_linkSequencer" {
          n209 = call "CAEObj.unfold trend data.vi"("i ref in"=w635, "raw trend data"=w633) -> ("quality"=w631:i32, "no link"=w639:bool, "data"=w638:i8[], "typeDescriptor"=w632:string, "error out"=w640:errorcluster)  [unwired: 9 in, 4 out]
          n210 = case shown="No Error" w640 {
            tunnel: [w663 w677] -> w636
            tunnel: w635 -> [w658 w677]
            tunnel: w634 -> [w660 w676]
            tunnel: [w661 w676] -> w637
            tunnel: w639 -> [w654 _]
            tunnel: w638 -> [w667 _]
            tunnel: w632 -> [w668 _]
            tunnel: w631 -> [w666 _]
            frame No Error {
              # "Das ist richtig!"
              n211 = call "PH_Timing.get i attribute.vi"("i ref in"=w658, "error in (no error)"=w660) -> ("i ref out"=w657:refnum<vi>, "i attribute"=w656:T8, "error out"=w659:errorcluster)  [unwired: 15 in]
              n212 = call "PH_DIM.get String.vi"("no link"=w654, "typeDescriptor"=w668, "data"=w667, "quality"=w666) -> ("Output String"=w665:string)
              n213 = Unbundle By Name(w656) -> ("Sequencer.linked?"=w655:bool)
              n214 = call "PH_Timing.PC link Sequencer.vi"("i ref in"=w657, "SM State"=w665, "no link"=w654, "error in"=w659) -> ("i ref out"=w651:refnum<vi>, "error out"=w649:errorcluster)  [unwired: 14 in]
              n215 = Bundle("linked?"=w655, "no link"=w654) -> (w653:cluster{"linked?":bool, "no link":bool})  [unwired: 1 in]
              n216 = Equal?(x=w653, y=cluster{"linked?":bool, "no link":bool} {"linked?"=FALSE, "no link"=FALSE}) -> (x = y?=w647:bool)
              n217 = case shown="True" w647 {
                tunnel: w651 -> [w670 w675]
                tunnel: [w670 w674] -> w650
                tunnel: w649 -> [w669 w673]
                tunnel: [w669 w672] -> w648
                frame False {
                }
                frame True {
                  n218 = call "PH_Timing.Action First Link Seq.vi"("i ref in"=w675, "Timing Mode"=T4 {"T2"=0, "Modeselector"=enum."Shot"}, "error IO"=w673) -> ("i ref out"=w674:refnum<vi>, "error out"=w672:errorcluster)  [unwired: 15 in]
                }
              }
              n219 = call "PH_Timing.Action link Sequencer.vi"("i ref in"=w650, "error in (no error)"=w648) -> ("i ref out"=w664:refnum<vi>, "error out"=w662:errorcluster)  [unwired: 16 in]
              n220 = call "PH_Timing.Update Status.vi"("i ref in"=w664, "error in (no error)"=w662) -> ("i ref out"=w663:refnum<vi>, "error out"=w661:errorcluster)  [unwired: 16 in]
            }
            frame Error {
            }
          }
          n221 = call "BaseProcess.set event status.vi"("i ref in"=w636, "EventStatus"=w641, "error in (no error)"=w637) -> ("i ref out"=w630:refnum<vi>, "error out"=w629:errorcluster)  [unwired: 14 in, 1 out]
          n222 = Unbundle By Name(w629) -> ("code"=w646:i32)
          n223 = case shown="No Error" w629 {
            selector: w629 -> [_ w681]
            tunnel: [T1 [] ("byteArray out") w680] -> w644
            frame No Error {
            }
            frame Error {
              n224 = Unbundle By Name(w681) -> ("source"=w679:string)
              n225 = call-poly "CoreLib.data 2 byte array.vi"("string"=w679) -> ("byteArray out"=w680:T1)  [unwired: 18 in]
            }
          }
          n226 = Bundle By Name(cluster=w642, "Data"=w644, "Error #"=w646, "Data Descriptor"="C:N") -> (w645:T2)
        }
        frame Default {
          n227 = call "PH_StatusHandler.ProcCases.vi"("i ref in"=w682, "selector"=w683, "Data"=w684, "call cluster"=w685, "error in (no error)"=w688) -> ("i ref out"=w689:refnum<vi>, "answer cluster"=w686:T2, "error out"=w687:errorcluster)  [unwired: 12 in]
        }
      }
    }
    frame Error {
    }
  }
  "answer cluster" <- w7
  "i ref out" <- w3
  "error out" <- w2
